vi "CreaInformeExcel.vi"(6 "Nom Assaig":string, 8 "NºTests":u8, 12 "Tabla":sgl[][](array[numeric])) -> (14 "status":bool, 19 "error out":errorcluster)   [LabVIEW 2017]
uses:
  <vilib>/addons/_office/excel.llb/Excel Easy Table (num).vi
  <vilib>/addons/_office/excel.llb/Excel Easy Table (str).vi
  <vilib>/Utility/NIReport.llb/NI_report.lvclass
  <vilib>/addons/_office/NI_ReportGenerationToolkit.lvlib
  <vilib>/Utility/NIReport.llb/Excel/NI_Excel.lvclass
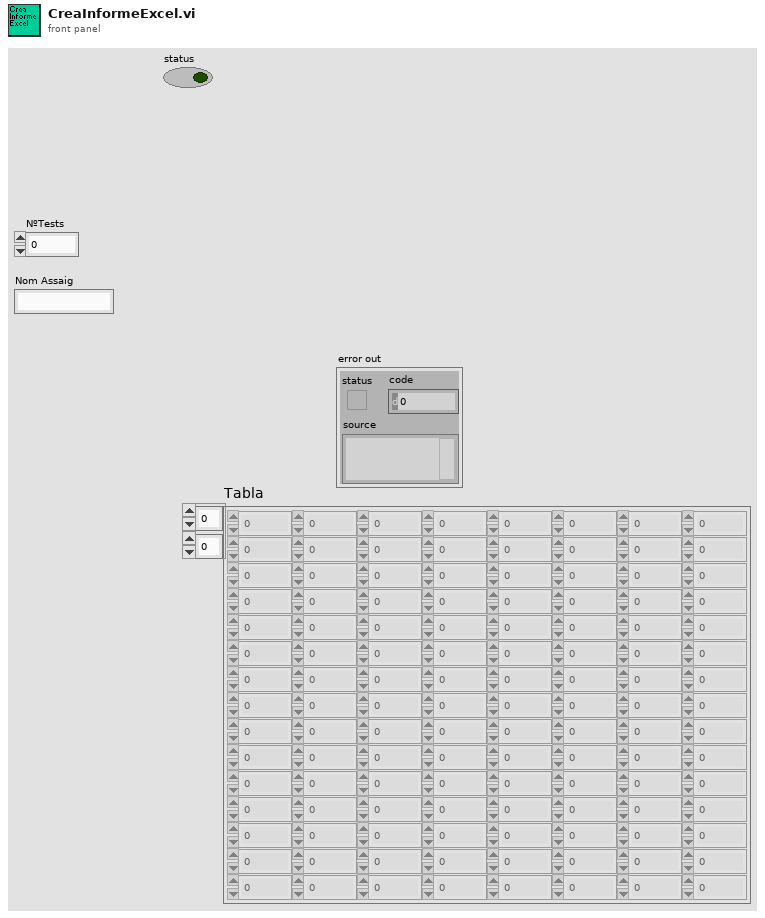
[diagram p1: front panel]
types:
  T1 = enum16{"maximized", "minimized", "normal", "no change"}
  T2 = enum16{"Standard Report", "HTML", "Word", "Excel"}
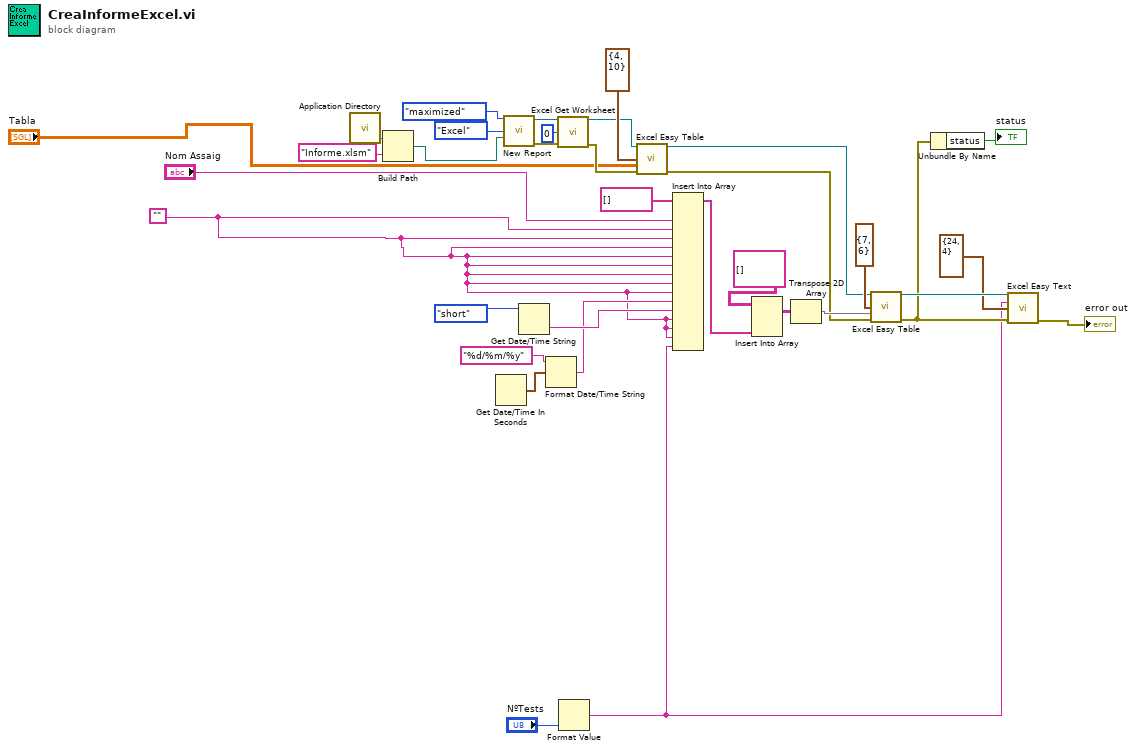
[diagram p0: block diagram]
diagram:
  w2 = ""
  n1 = call <vilib>:"Application Directory.vi"() -> ("Application Directory"=w19:path)
  n2 = Build Path(base path=w19, name or relative path="Informe.xlsm") -> (appended path=w21:path)
  n3 = Get Date/Time In Seconds() -> (seconds since 1Jan1904=w14:timestamp)
  n4 = call <vilib>:"New Report.vi"("window state (normal)"=T1."maximized", "report type"=T2."Excel", "template (empty)"=w21) -> ("report out"=w12:refnum<class "NI_report.lvclass">, "error out"=w9:errorcluster)  [unwired: 11 in]
  n5 = Get Date/Time String(date format (0)=enum16{"short", "long", "abbreviated"}."short") -> (time string=w17:string)  [unwired: 2 in, 1 out]
  n6 = Format Date/Time String(time format string (%c)="%d/%m/%y", seconds (now)=w14) -> (date/time string=w13:string)  [unwired: 1 in]
  n7 = call <vilib>:"Excel Get Worksheet.vi"("report in"=w12, "worksheet index (0)"=0, "error in (no error)"=w9) -> ("report out"=w11:refnum<class "NI_report.lvclass">, "error out"=w8:errorcluster)  [unwired: 11 in]
  n8 = Format Value(value (0)="NºTests") -> (output string=w4:string)  [unwired: 2 in]
  n9 = call-poly <vilib>:"Excel Easy Table.vi"("report in"=w11, "start (0, 0)"=cluster{"row":i32, "column":i32} {"row"=4, "column"=10}, "text data"="Tabla", "error in (no error)"=w8) -> ("report out"=w25:refnum<class "NI_report.lvclass">, "error out"=w26:errorcluster)  [unwired: 7 in, 3 out]
  n10 = Insert Into Array(array=string[] [] ("new element/subarray"), new element #1="Nom Assaig", new element #2=w2, new element #3=w2, new element #4=w2, new element #5=w2, new element #6=w2, new element #7=w2, new element #8=w2, new element #9=w2, new element #10=w13, new element #11=w17, new element #12=w2, new element #13=w2, new element #14=w2, new element #15=w4) -> (w30:string[])  [unwired: 1 in]
  n11 = Insert Into Array(array=string[][] [] ("text data"), new element=w30) -> (w32:string[][])  [unwired: 2 in]
  n12 = Transpose 2D Array(2D array=w32) -> (transposed array=w31:string[][])
  n13 = call-poly <vilib>:"Excel Easy Table.vi"("report in"=w25, "start (0, 0)"=cluster{"row":i32, "column":i32} {"row"=7, "column"=6}, "text data"=w31, "error in (no error)"=w26) -> ("report out"=w7:refnum<class "NI_report.lvclass">, "error out"=w6:errorcluster)  [unwired: 7 in, 3 out]
  n14 = Unbundle By Name(w6) -> ("status"=→"status":bool)
  n15 = call <vilib>:"Excel Easy Text.vi"("report in"=w7, "text"=w4, "start (-1, -1)"=cluster{"row":i32, "column":i32} {"row"=24, "column"=4} ("start (0, 0)"), "error in (no error)"=w6) -> ("error out"=→"error out":errorcluster)  [unwired: 7 in, 4 out]
